vi "myRIO__TCP_disconnect_forRead.vi"(8 "input_error":errorcluster, 11 "input_hTCP":refnum<k5>) -> (0 "output_error":errorcluster)   [LabVIEW 2014]
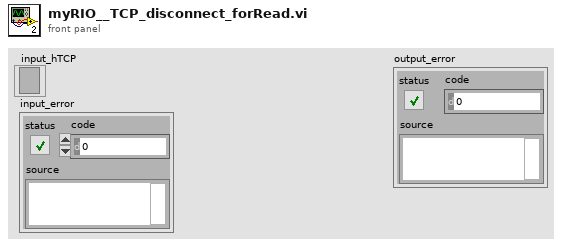
[diagram p1: front panel]
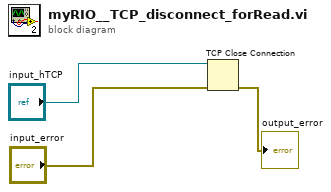
[diagram p0: block diagram]
diagram:
  n1 = TCP Close Connection(connection ID="input_hTCP", error in (no error)="input_error") -> (error out=→"output_error":errorcluster)  [unwired: 1 in, 1 out]
